vi "Sql_datetime format.vi"(8 "error in (no error)":errorcluster, 11 "Date time In":string) -> (0 "error out":errorcluster, 3 "Sql datetime type 20":string)   [LabVIEW 2013]
panel:
  out "Array":string[](array[string])
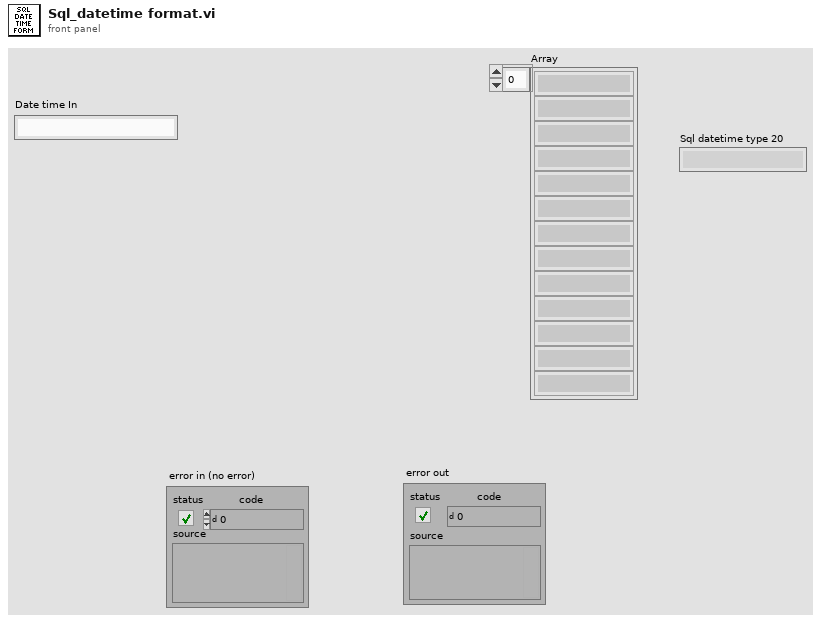
[diagram p1: front panel]
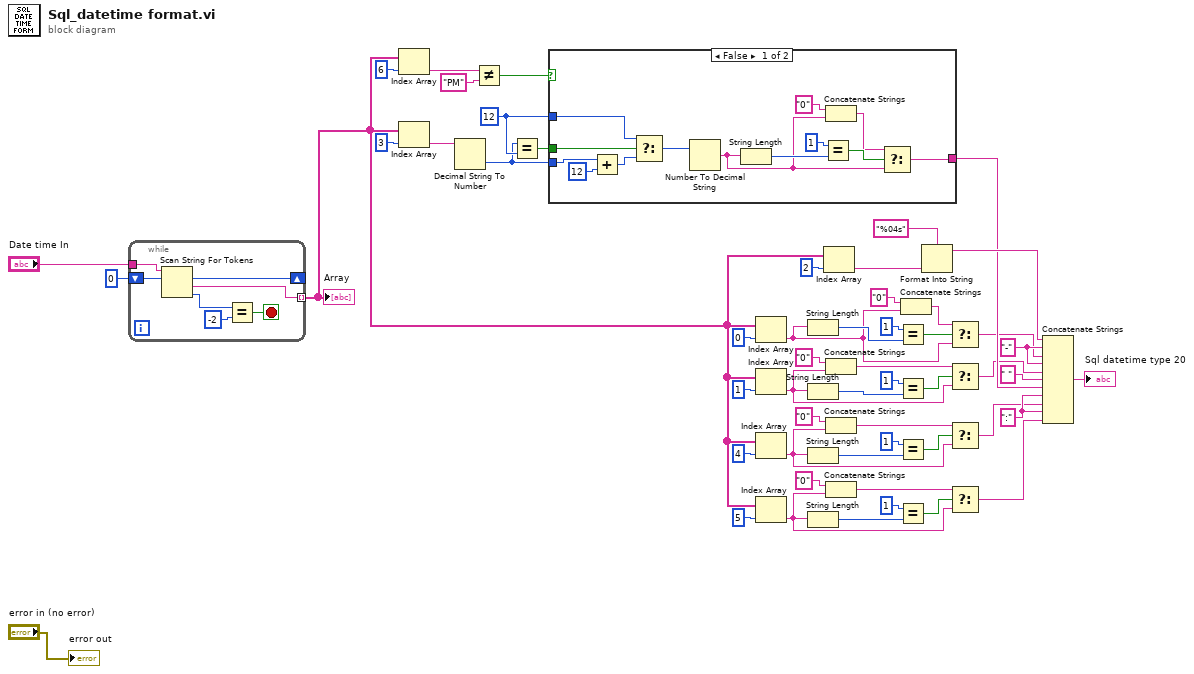
[diagram p0: block diagram]
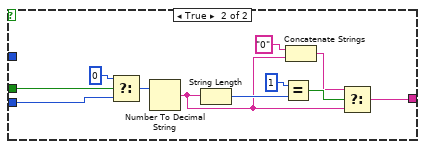
[diagram p2: hidden frame]
diagram:
  w31 = ":" ("string")
  w35 = "-" ("string")
  w37 = 12 ("y")
  n1 = while {
    tunnel: "Date time In" -> [w61]
    shift-right: [w57] -> _
    shift-left: 0 -> [w58]
    tunnel: [w55] -> w42 mode=indexing
    stop <- w59 stop-if-true
    n2 = Scan String For Tokens(8:w58, 9:w61) -> (0:w56:i32, 1:w55:string, 2:w57:i32)  [unwired: 4 in, 1 out]
    n3 = Equal?(x=w56, y=-2) -> (x = y?=w59:bool)
  }
  "Array" <- w42
  n4 = Index Array(array=w42, index=6) -> (element=w41:string)
  n5 = Index Array(array=w42, index=3) -> (element=w44:string)
  n6 = Decimal String To Number(string=w44) -> (number=w2:i32)  [unwired: 2 in, 1 out]
  n7 = Not Equal?(x=w41, y="PM") -> (x != y?=w39:bool)
  n8 = Equal?(x=w2, y=w37) -> (x = y?=w38:bool)
  n9 = case shown="False" w39 {
    tunnel: w38 -> [w74 w85]
    tunnel: w37 -> [w72 _]
    tunnel: [w63 w75] -> w33
    tunnel: w2 -> [w70 w83]
    frame False {
      n10 = Add(x=w70, y=12) -> (x+y=w73:i32)
      n11 = Select(t=w72, s=w74, f=w73) -> (s? t:f=w62:i32)
      n12 = Number To Decimal String(number=w62) -> (decimal integer string=w64:string)  [unwired: 1 in]
      n13 = String Length(string=w64) -> (length=w69:i32)
      n14 = Equal?(x=1, y=w69) -> (x = y?=w67:bool)
      n15 = Concatenate Strings("0" ("format string"), w64) -> (w65:string)
      n16 = Select(t=w65, s=w67, f=w64) -> (s? t:f=w63:string)
    }
    frame True {
      n17 = Select(t=i16 0 ("width (-)"), s=w85, f=w83) -> (s? t:f=w82:i32)
      n18 = Number To Decimal String(number=w82) -> (decimal integer string=w76:string)  [unwired: 1 in]
      n19 = String Length(string=w76) -> (length=w81:i32)
      n20 = Equal?(x=1, y=w81) -> (x = y?=w79:bool)
      n21 = Concatenate Strings("0" ("format string"), w76) -> (w77:string)
      n22 = Select(t=w77, s=w79, f=w76) -> (s? t:f=w75:string)
    }
  }
  n23 = Index Array(array=w42, index=0) -> (element=w25:string)
  n24 = Index Array(array=w42, index=1) -> (element=w18:string)
  n25 = Index Array(array=w42, index=4) -> (element=w11:string)
  n26 = Index Array(array=w42, index=5) -> (element=w4:string)
  n27 = String Length(string=w25) -> (length=w30:i32)
  n28 = String Length(string=w18) -> (length=w19:i32)
  n29 = String Length(string=w11) -> (length=w16:i32)
  n30 = String Length(string=w4) -> (length=w5:i32)
  n31 = Index Array(array=w42, index=2) -> (element=w48:string)
  n32 = Concatenate Strings("0" ("format string"), w18) -> (w23:string)
  n33 = Concatenate Strings("0" ("format string"), w11) -> (w12:string)
  n34 = Concatenate Strings("0" ("format string"), w4) -> (w9:string)
  n35 = Equal?(x=1, y=w30) -> (x = y?=w28:bool)
  n36 = Equal?(x=1, y=w19) -> (x = y?=w21:bool)
  n37 = Equal?(x=1, y=w16) -> (x = y?=w14:bool)
  n38 = Equal?(x=1, y=w5) -> (x = y?=w7:bool)
  n39 = Concatenate Strings("0" ("format string"), w25) -> (w26:string)
  n40 = Format Into String(format string="%04s", w48) -> (resulting string=w36:string)  [unwired: 2 in, 1 out]
  n41 = Select(t=w26, s=w28, f=w25) -> (s? t:f=w24:string)
  n42 = Select(t=w23, s=w21, f=w18) -> (s? t:f=w17:string)
  n43 = Select(t=w12, s=w14, f=w11) -> (s? t:f=w10:string)
  n44 = Select(t=w9, s=w7, f=w4) -> (s? t:f=w3:string)
  n45 = Concatenate Strings(w36, w35, w24, w35, w17, " " ("string"), w33, w31, w10, w31, w3) -> (→"Sql datetime type 20":string)
  "error out" <- "error in (no error)"
